vi "Pre Launch Init.vi"(11 "Limites Contador in":refnum<class "Limites Contador.lvclass">) -> (0 "error out":errorcluster, 3 "Limites Contador out":refnum<class "Limites Contador.lvclass">)   [LabVIEW 2020, in "Limites Contador.lvlib" / "Limites Contador.lvclass"]
doc: "(<B>Filename</B>: Actor Framework.lvlib:Actor.lvclass:Pre Launch Init.vi)\n\nDefines behavior that occurs after the Launch Nested Actor method is invoked but before the actor's Actor Core method begins running.\n\nBy default, this method does nothing. A descendant class may override it to define behavior."
uses:
  Limites Contador.lvclass
  <vilib>/ActorFramework/Actor/Actor.lvclass
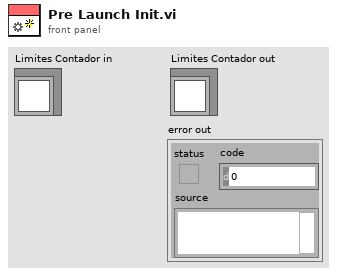
[diagram p1: front panel]
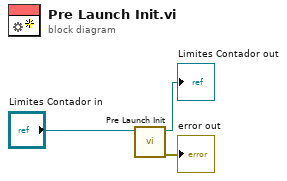
[diagram p0: block diagram]
diagram:
  n1 = call-parent "Pre Launch Init.vi"("Actor in"="Limites Contador in") -> ("error out"=→"error out":errorcluster, "Actor out"=→"Limites Contador out":refnum<class "Limites Contador.lvclass">)  [unwired: 9 in]
